vi "Write Address.vi"(8 "error in":errorcluster, 10 "Address":string, 11 "TCP master in":refnum<class "TCP Interface.lvclass">) -> (0 "error out":errorcluster, 3 "TCP master out":refnum<class "TCP Interface.lvclass">)   [LabVIEW 2021, in "TCP Interface.lvclass"]
doc: "Property accessor for the TCP address."
uses:
  TCP Interface.lvclass
  TCP Interface.lvclass/TCP Interface.ctl
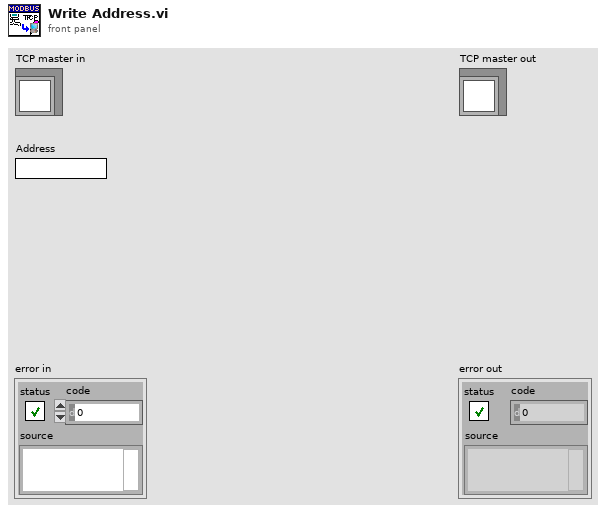
[diagram p1: front panel]
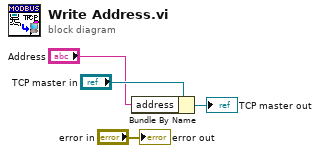
[diagram p0: block diagram]
diagram:
  n1 = Bundle By Name(cluster="TCP master in", "address"="Address") -> (→"TCP master out":refnum<class "TCP Interface.lvclass">)
  "error out" <- "error in"
